vi "move_backward.vi"(5 "core_data in":T1) -> (0 "tour in progress":T3[](array[typedef]), 1 "chessboard":T4[][](array[typedef]), 2 "core_data out":T1)   [LabVIEW 2020, in "core.lvlib"]
uses:
  core.lvlib
  core_data/chess_square.ctl
  core_data/neighbour_square.ctl
  core_data/chessboard_index.ctl
  core_data/core_data.ctl
  core_data/tour_in_progress.ctl
  core_data/library_variable.vi
  core_data/core_data.lvlib
panel:
  # "Development\ncontrols/indicators useful for development and testing, but which are not outputs of the VI"
  # "Input\nInputs to the VI"
  # "Output\nOutputs of the VI"
  # "Description\n\nBlank VI with error handling case. \n\nSummarize the use of this VI in this space."
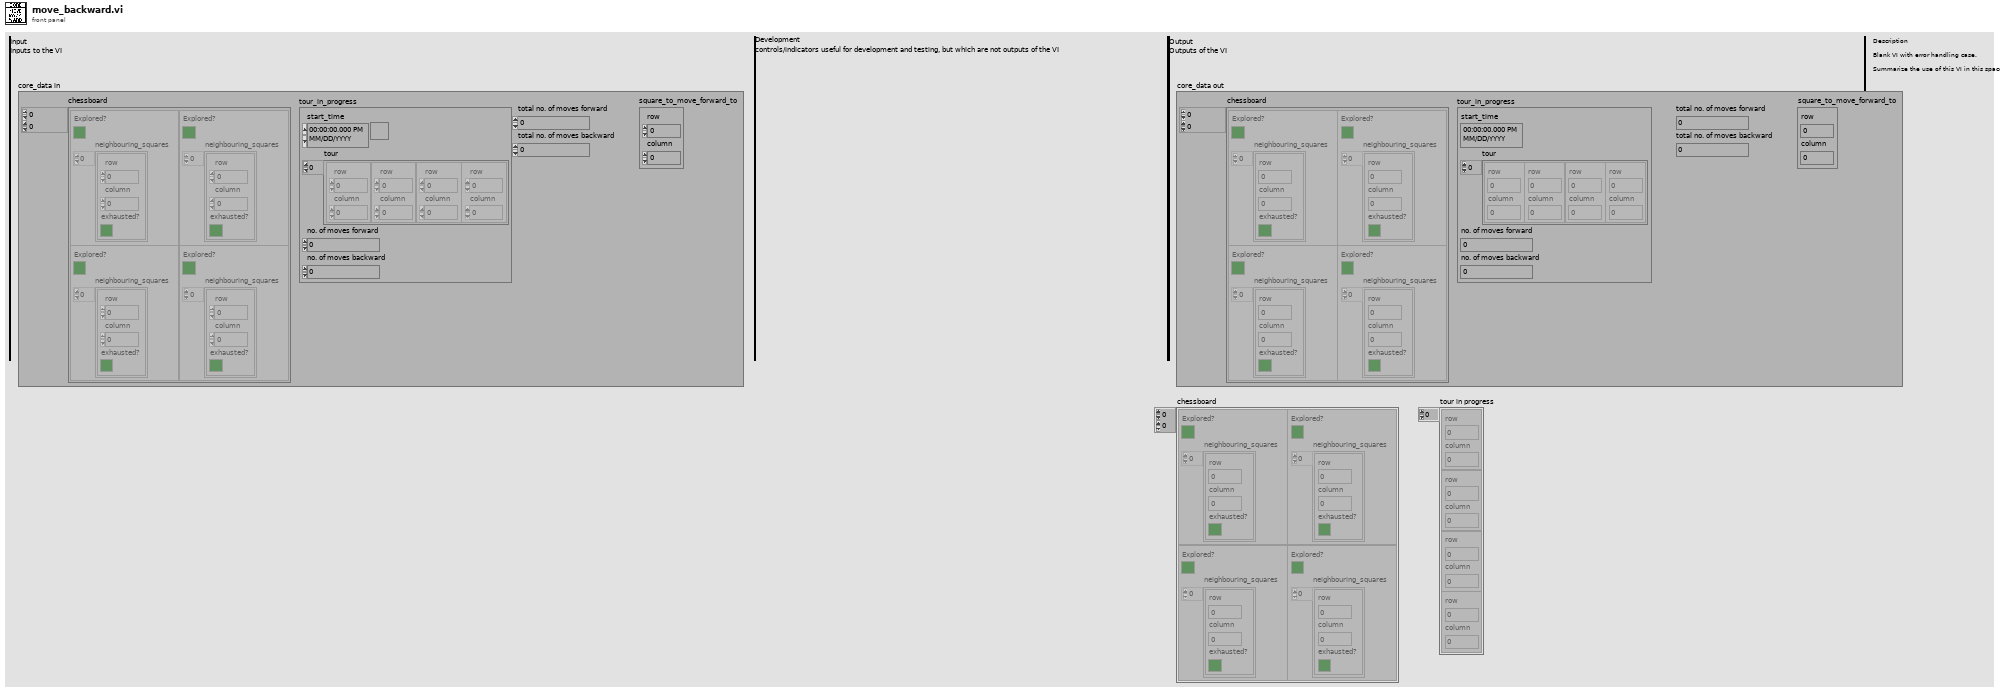
[diagram p1: front panel]
types:
  T1 = typedef "core.lvlib/core_data.lvlib/core_data.ctl" = cluster{"tour_in_progress":T2, "total no. of moves forward":u64, "total no. of moves backward":u64, "chessboard":T4[][], "square_to_move_forward_to":T3}
  T2 = typedef "core.lvlib/core_data.lvlib/tour_in_progress.ctl" = cluster{"start_time":timestamp, "tour":T3[], "no. of moves forward":u64, "no. of moves backward":u64}
  T3 = typedef "core.lvlib/core_data.lvlib/chessboard_index.ctl" = cluster{"row":u8, "column":u8}
  T4 = typedef "core.lvlib/core_data.lvlib/chess_square.ctl" = cluster{"Explored?":bool, "neighbouring_squares":T5[]}
  T5 = typedef "core.lvlib/core_data.lvlib/neighbour_square.ctl" = cluster{"row":u8, "column":u8, "exhausted?":bool}
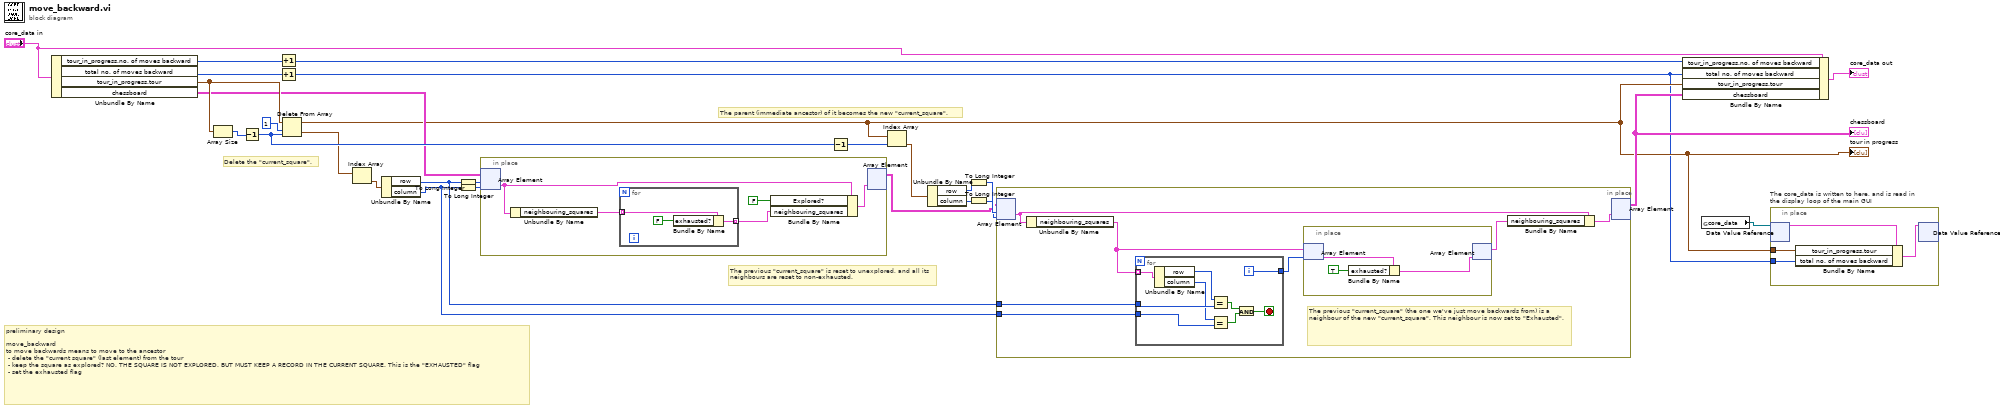
[diagram p0: block diagram]
diagram:
  # "The previous \"current_square\" is reset to unexplored, and all its neighbours are reset to non-exhausted."
  # "The parent (immediate ancestor) of it becomes the new \"current_square\"."
  # "Delete the \"current_square\"."
  # "preliminary design\n\nmove_backward\nto move backwards means to move to the ancestor\n - delete the \"current square\" (last element) from the tour\n - keep the square as explored? NO. THE SQUARE IS NOT EXPLORED. BUT MUST KEEP A RECORD IN THE CURRENT SQUARE. This is the \"EXHAUSTED\" flag\n - set the exhausted flag"
  n1 = Unbundle By Name("core_data in") -> ("tour_in_progress.no. of moves backward"=w7:u64, "total no. of moves backward"=w24:u64, "tour_in_progress.tour"=w23:T3[], "chessboard"=w17:T4[][])
  n2 = Array Size(array=w23) -> (size(s)=w22:i32)
  n3 = Decrement(x=w22) -> (x-1=w20:i32)
  n4 = Increment(x=w7) -> (x+1=w6:u64)
  n5 = Increment(x=w24) -> (x+1=w4:u64)
  n6 = Delete From Array "Delete From Array"(array=w23, length=1, index=w20) -> (deleted portion=w2:T3[], array with subset deleted=w5:T3[])
  "tour in progress" <- w5
  n7 = Index Array(array=w2) -> (element=w18:T3)  [unwired: 1 in]
  n8 = Unbundle By Name(w18) -> ("row"=w9:u8, "column"=w8:u8)
  n9 = To Long Integer(number=w9) -> (32bit integer=w16:i32)
  n10 = To Long Integer(number=w8) -> (32bit integer=w15:i32)
  n11 = in-place {
    n12 = in-place-array #1(w17, w16, w15) -> (w30:T4)
    n13 = Unbundle By Name(w30) -> ("neighbouring_squares"=w29:T5[])
    n14 = for {
      tunnel: w29 -> [w35] mode=indexing
      tunnel: [w33] -> w28 mode=indexing
      n15 = Bundle By Name(cluster=w35, "exhausted?"=FALSE) -> (w33:T5)
    }
    n16 = Bundle By Name(cluster=w30, "Explored?"=FALSE, "neighbouring_squares"=w28) -> (w31:T4)
    n17 = in-place-array #1(w31) -> (w1:T4[][])  [unwired: 2 out]
  }
  n18 = Decrement(x=w20) -> (x-1=w19:i32)
  n19 = Index Array(array=w5, index=w19) -> (element=w14:T3)
  n20 = Unbundle By Name(w14) -> ("row"=w13:u8, "column"=w12:u8)
  n21 = To Long Integer(number=w13) -> (32bit integer=w11:i32)
  n22 = To Long Integer(number=w12) -> (32bit integer=w10:i32)
  n23 = in-place {
    in-place-border: w9 -> [w38]
    in-place-border: w8 -> [w37]
    # "The previous \"current_square\" (the one we've just move backwards from) is a neighbour of the new \"current_square\". This neighbour is now set to \"Exhausted\"."
    n24 = in-place-array #2(w1, w11, w10) -> (w42:T4)
    n25 = Unbundle By Name(w42) -> ("neighbouring_squares"=w39:T5[])
    n26 = for {
      tunnel: w39 -> [w51] mode=indexing
      tunnel: w38 -> [w49]
      tunnel: w37 -> [w47]
      tunnel: [w43] -> w36
      i -> [w43]
      stop <- w44 stop-if-true
      n27 = Unbundle By Name(w51) -> ("row"=w50:u8, "column"=w48:u8)
      n28 = Equal?(x=w50, y=w49) -> (x = y?=w46:bool)
      n29 = Equal?(x=w48, y=w47) -> (x = y?=w45:bool)
      n30 = And(x=w46, y=w45) -> (x .and. y?=w44:bool)
    }
    n31 = in-place {
      n32 = in-place-array #3(w39, w36) -> (w54:T5)
      n33 = Bundle By Name(cluster=w54, "exhausted?"=TRUE) -> (w52:T5)
      n34 = in-place-array #3(w52) -> (w41:T5[])  [unwired: 1 out]
    }
    n35 = Bundle By Name(cluster=w42, "neighbouring_squares"=w41) -> (w40:T4)
    n36 = in-place-array #2(w40) -> (w27:T4[][])  [unwired: 2 out]
  }
  "chessboard" <- w27
  n37 = Bundle By Name(cluster="core_data in", "tour_in_progress.no. of moves backward"=w6, "total no. of moves backward"=w4, "tour_in_progress.tour"=w5, "chessboard"=w27) -> (→"core_data out":T1)
  n38 = global read "library_variable.vi" "core_data"() -> (w3:refnum<data-value>)
  n39 = in-place "The core_data is written to here, and is read in the display loop of the main GUI" {
    in-place-border: w5 -> [w56]
    in-place-border: w4 -> [w55]
    n40 = in-place-dvr #4(w3) -> (w58:T1)  [unwired: 1 out]
    n41 = Bundle By Name(cluster=w58, "tour_in_progress.tour"=w56, "total no. of moves backward"=w55) -> (w57:T1)
    n42 = in-place-dvr #4(w57) -> ()  [unwired: 2 out]
  }
